vi "AddIndexs.vi"(8 "error in (no error)":errorcluster, 11 "List in":refnum<class "List.lvclass">) -> (0 "error out":errorcluster, 3 "List out":refnum<class "List.lvclass">)   [LabVIEW 2015, in "List.lvclass"]
uses:
  List.lvclass
  List.lvclass/List.ctl
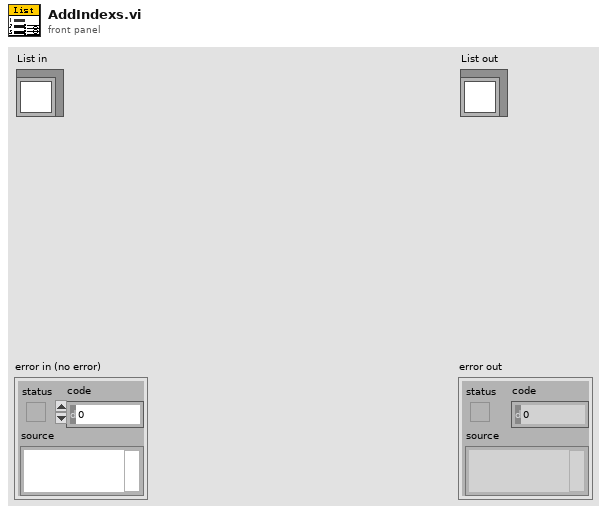
[diagram p1: front panel]
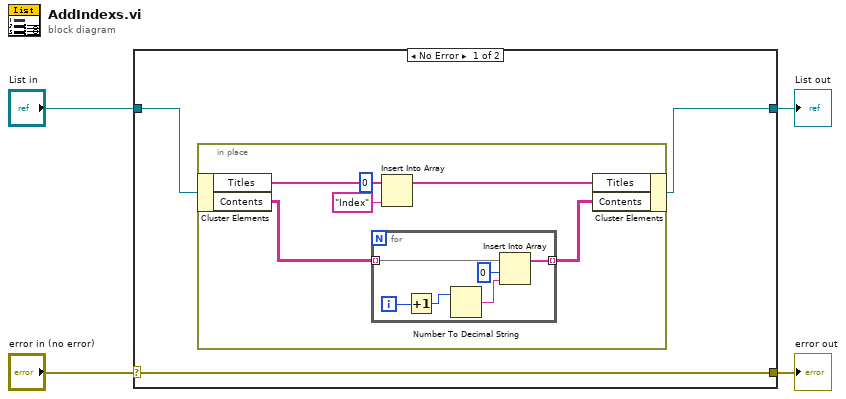
[diagram p0: block diagram]
diagram:
  n1 = case shown="No Error" "error in (no error)" {
    selector: "error in (no error)" -> [w7 w21]
    tunnel: [w7 w21] -> w3
    tunnel: [w5 w20] -> w1
    tunnel: "List in" -> [w6 w20]
    frame No Error {
      n2 = in-place {
        n3 = in-place-cluster #1(w6) -> ("Titles"=w13:string[], "Contents"=w9:string[][])
        n4 = for {
          tunnel: w9 -> [w19] mode=indexing
          tunnel: [w14] -> w8 mode=indexing
          i -> [w18]
          n5 = Increment(x=w18) -> (x+1=w17:i32)
          n6 = Number To Decimal String(number=w17) -> (decimal integer string=w16:string)  [unwired: 1 in]
          n7 = Insert Into Array(array=w19, index=0, new element=w16) -> (w14:string[])
        }
        n8 = Insert Into Array(array=w13, index=0, new element="Index" ("new element/subarray")) -> (w11:string[])
        n9 = in-place-cluster #1("Titles"=w11, "Contents"=w8) -> (w5:refnum<class "List.lvclass">)
      }
    }
    frame Error {
    }
  }
  "error out" <- w3
  "List out" <- w1
